vi "utime_sleep_us.vi"(9 "wait (µs)":u32, 11 "Data In":T1) -> (3 "Data Out":T1={"Port"="", "All Code"="Hi"})   [LabVIEW 2016]
uses:
  uPythonX/PythonData.ctl
  uPythonX/uPythonX.xctl
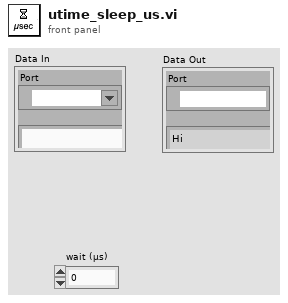
[diagram p1: front panel]
types:
  T1 = typedef "uPythonX.xctl/PythonData.ctl" = cluster{"Port":refnum<visa-resource-name>, "All Code":string}
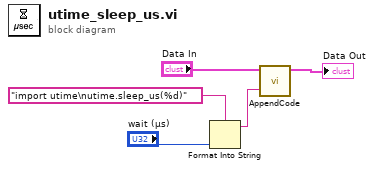
[diagram p0: block diagram]
diagram:
  n1 = Format Into String(format string="import utime\nutime.sleep_us(%d)", "wait (µs)") -> (resulting string=w1:string)  [unwired: 2 in, 1 out]
  n2 = call "AppendCode.vi"("New Code"=w1, "Data In"="Data In") -> ("Data Out"=→"Data Out":T1)  [unwired: 9 in]
